vi "SetPaneOriginToPaneInstance.vi"(7 "Pane number":u16, 8 "error in (no error)":errorcluster, 9 "Panes Origin differ by - X(T) or Y(F)":bool=TRUE, 10 "Pane":u16(ring) items=["Top", "Left", "Center", "Right", "Bottom"], 11 "PentaPanesGUI in":refnum<class "PentaPanes.lvclass">) -> (0 "error out":errorcluster, 3 "PentaPanesGUI out":refnum<class "PentaPanes.lvclass">)   [LabVIEW 2022 SP3, in "PentaPanesLibrary.lvlib" / "PentaPanes.lvclass"]
doc: "SetPaneOriginToPaneInstance. \nIn case of multiple pane instances this VI sets the pane origin to the correct Pane instance to be shown. \n\nPane - The pane that contains the multiple pane instances \nPane number - the number of the instance to show. \nPanes Origin differ by - Choose if the pane instances are seperated by X or Y axis"
uses:
  PentaPanes.lvclass
  <vilib>/Utility/miscctls.llb/LVBoundsTypeDef.ctl
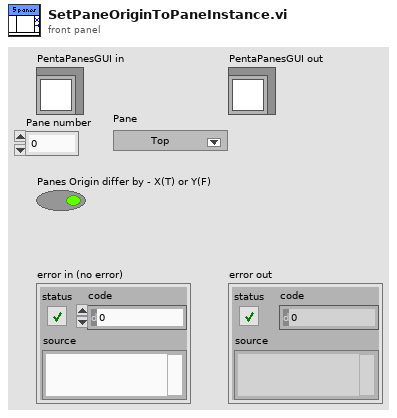
[diagram p1: front panel]
types:
  T1 = typedef "LVBoundsTypeDef.ctl" = cluster{"Width":i32, "Height":i32}
  T2 = typedef "LVBoundsTypeDef.ctl" = cluster{"Width":u32, "Height":u32}
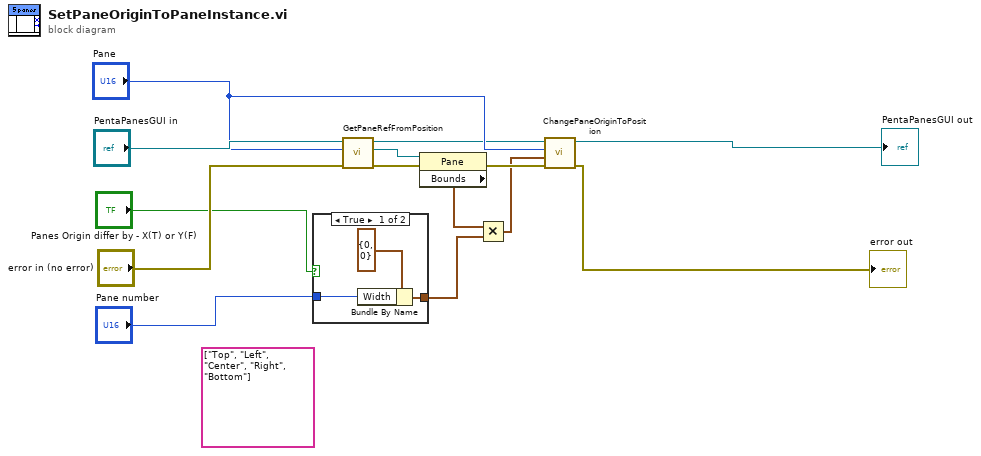
[diagram p0: block diagram]
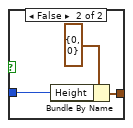
[diagram p2: hidden frame]
diagram:
  (unwired) string[] ["Top", "Left", "Center", "Right", "Bottom"]
  n1 = case shown="True" "Panes Origin differ by - X(T) or Y(F)" {
    tunnel: [w16 w19] -> w2
    tunnel: "Pane number" -> [w15 w18]
    frame True {
      n2 = Bundle By Name(cluster=T1 {"Width"=0, "Height"=0} ("Bounds"), "Width"=w15) -> (w16:T1)
    }
    frame False {
      n3 = Bundle By Name(cluster=T1 {"Width"=0, "Height"=0} ("Bounds"), "Height"=w18) -> (w19:T1)
    }
  }
  n4 = call "GetPaneRefFromPosition.vi"("error in (no error)"="error in (no error)", "Position"="Pane", "PentaPanesGUI in"="PentaPanesGUI in") -> ("error out"=w11:errorcluster, "PaneRef"=w13:refnum<vi>, "PentaPanesGUI out"=w8:refnum<class "PentaPanes.lvclass">)  [unwired: 6 in]
  n5 = property class="Pane"(reference=w13, error in=w11) -> (error out=w7:errorcluster, "Bounds"=w3:T2)  [unwired: 1 out]
  n6 = Multiply(x=w3, y=w2) -> (x*y=w1:T2)
  n7 = call "ChangePaneOriginToPosition.vi"("error in (no error)"=w7, "New Origin"=w1, "Pane"="Pane", "PentaPanesGUI in"=w8) -> ("error out"=→"error out":errorcluster, "PentaPanesGUI out"=→"PentaPanesGUI out":refnum<class "PentaPanes.lvclass">)  [unwired: 6 in]
